vi "PCO_GetMaxNumberOfImagesInSegment.vi"(8 "error in (no error)":errorcluster {"code" format="%x"}, 11 "ph":u64) -> (0 "error out":errorcluster {"code" format="%x"}, 1 "dwMaxNumberImages":u32, 2 "ErrorMessage":i32 format="%x", 3 "ph out":u64)   [LabVIEW 2019, in "SDK.lvlib" / "StorageControl.lvlib"]
doc: "<b>Description:</b>\nGets the maximum number of images in active segment.\n\n<b>Supported camera type:</b>\npco.dimax, pco.1200, pco.1600, pco.2000, pco.4000\n\n<b>Descriptor dependency:</b>\ndwGeneralCapsDESC1: NO_RECORDER"
uses:
  StorageControl.lvlib
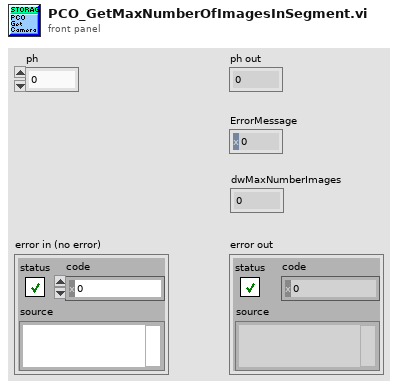
[diagram p1: front panel]
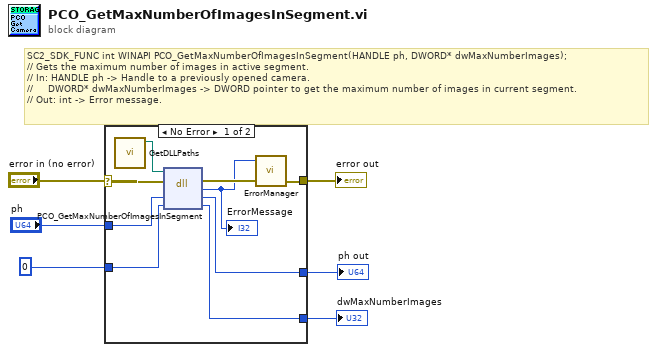
[diagram p0: block diagram]
diagram:
  # "SC2_SDK_FUNC int WINAPI PCO_GetMaxNumberOfImagesInSegment(HANDLE ph, DWORD* dwMaxNumberImages);\n// Gets the maximum number of images in active segment.\n// In: HANDLE ph -> Handle to a previously opened camera.\n//     DWORD* dwMaxNumberImages -> DWORD pointer to get the maximum number of images in current segment.\n// Out: int -> Error message."
  n1 = case shown="No Error" "error in (no error)" {
    selector: "error in (no error)" -> [w11 w18]
    tunnel: "ph" -> [w15 w17]
    tunnel: [w14 w17] -> w5
    tunnel: [w9 w18] -> w4
    tunnel: [w13 w16] -> w3
    tunnel: u32 0 ("dwRamSegSize") -> [w12 w16]
    frame No Error {
      n2 = call "GetDLLPaths.vi"() -> ("SC2_Cam_Path"=w7:path)  [unwired: 9 in, 2 out]
      n3 = dll-call lib="?" fn="PCO_GetMaxNumberOfImagesInSegment"(path in=w7, error in=w11, "ph"=w15, "dwMaxNumberImages"=w12) -> (error out=w10:errorcluster, "return type"=w8:i32, "ph"=w14:u64, "dwMaxNumberImages"=w13:u32)  [unwired: 1 in, 1 out]
      "ErrorMessage" <- w8
      n4 = call "ErrorManager.vi"("error in (no error)"=w10, "error code"=w8) -> ("error out"=w9:errorcluster)  [unwired: 3 in]
    }
    frame Error {
    }
  }
  "ph out" <- w5
  "error out" <- w4
  "dwMaxNumberImages" <- w3
